vi "verify #frames.vi"(8 "error in (no error)":errorcluster, 11 "Simulated_CCD_Camera in":refnum<class "Sim_Ixon_Ultra.lvclass">) -> (0 "error out":errorcluster, 3 "Simulated_CCD_Camera out":refnum<class "Sim_Ixon_Ultra.lvclass">)   [LabVIEW 2018, in "Sim_Ixon_Ultra.lvclass"]
doc: "Verify the related parameters of the camera\n\nThere are some parameters of the camera operation mode that depend on the value provided for another parameter. This function verifies if these parameters are in agreement."
uses:
  Sim_Ixon_Ultra.lvclass
  <vilib>/ErrorRing/Error Ring.xnode
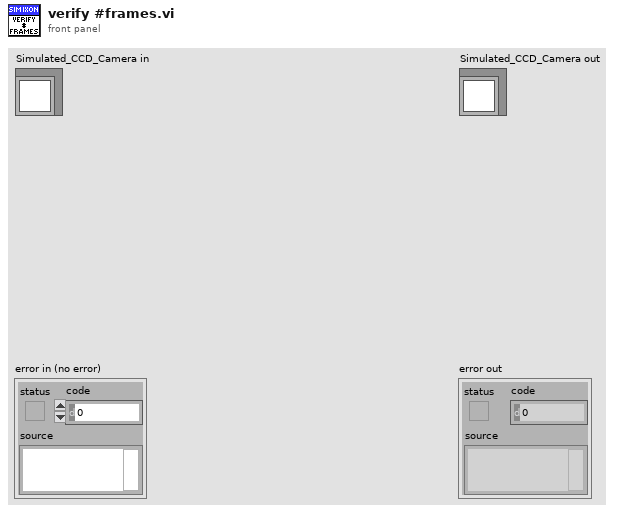
[diagram p1: front panel]
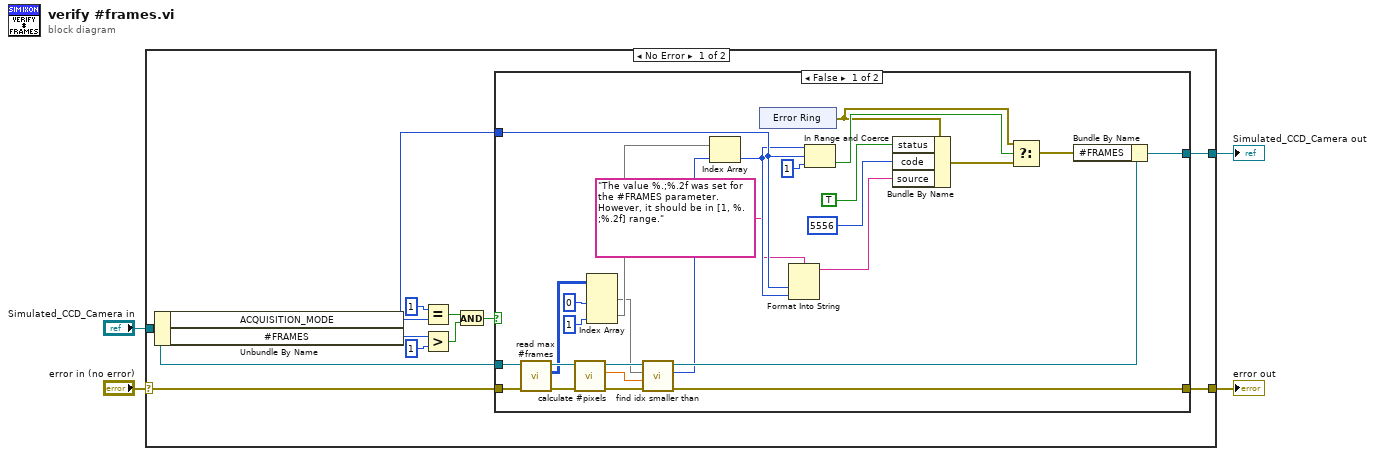
[diagram p0: block diagram]
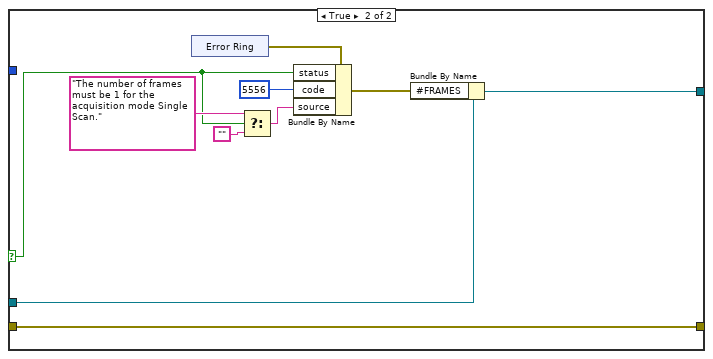
[diagram p2: hidden frame]
diagram:
  n1 = case shown="No Error" "error in (no error)" {
    selector: "error in (no error)" -> [w11 w56]
    tunnel: [w8 w56] -> w3
    tunnel: [w9 w55] -> w1
    tunnel: "Simulated_CCD_Camera in" -> [w10 w55]
    frame No Error {
      n2 = Unbundle By Name(w10) -> ("ACQUISITION_MODE"=w6:u16, "#FRAMES"=w5:u32)
      n3 = Equal?(x=u16 1, y=w6) -> (x = y?=w13:bool)
      n4 = Greater?(x=w5, y=1) -> (0:w14:bool)
      n5 = And(x=w13, y=w14) -> (x .and. y?=w7:bool)
      n6 = case shown="False" w7 {
        selector: w7 -> [_ w44]
        tunnel: [w33 w51] -> w9
        tunnel: w10 -> [w41 w52]
        tunnel: w11 -> [w42 w50]
        tunnel: [w29 w50] -> w8
        tunnel: w5 -> [w32 _]
        frame False {
          n7 = call "read max #frames.vi"("error in (no error)"=w42, "Simulated_CCD_Camera in"=w41) -> ("error out"=w40:errorcluster, "max #pix"=w38:i64[][], "Simulated_CCD_Camera out"=w39:refnum<class "Sim_Ixon_Ultra.lvclass">)  [unwired: 7 in]
          n8 = call "calculate #pixels.vi"("error in (no error)"=w40, "Simulated Camera in"=w39) -> ("error out"=w30:errorcluster, "#pixels"=w25:dbl, "Simulated Camera out"=w27:refnum<class "Sim_Ixon_Ultra.lvclass">)  [unwired: 7 in]
          n9 = Index Array(array=w38, index (col) #1=0 ("disabled index (col)"), index (col) #2=1 ("disabled index (col)")) -> (element #1=w26:i64[], element #2=w35:i64[])  [unwired: 2 in]
          n10 = call "find idx smaller than.vi"("error in (no error)"=w30, "Numeric"=w25, "Array"=w26, "Simulated Camera in"=w27) -> ("error out"=w29:errorcluster, "index"=w24:i32, "Simulated Camera out"=w28:refnum<class "Sim_Ixon_Ultra.lvclass">)  [unwired: 5 in]
          n11 = Index Array(array=w35, index=w24) -> (element=w31:i64)
          n12 = xnode "Error Ring"() -> ("error out"=w16:errorcluster)
          n13 = Format Into String(format string="The value %.;%.2f was set for the #FRAMES parameter. However, it should be in [1, %.;%.2f] range." ("string"), w32, w31) -> (resulting string=w21:string)  [unwired: 2 in, 1 out]
          n14 = In Range and Coerce(upper limit=w31, x=w32, lower limit=1) -> (In Range?=w19:bool)  [unwired: 1 out]
          n15 = Bundle By Name(cluster=w16, "status"=TRUE, "code"=5556, "source"=w21) -> (w17:errorcluster)
          n16 = Select(t=w16, s=w19, f=w17) -> (s? t:f=w18:errorcluster)
          n17 = Bundle By Name(cluster=w28, "#FRAMES"=w18) -> (w33:refnum<class "Sim_Ixon_Ultra.lvclass">)
        }
        frame True {
          n18 = xnode "Error Ring"() -> ("error out"=w53:errorcluster)
          n19 = Select(t="The number of frames must be 1 for the acquisition mode Single Scan.", s=w44, f="") -> (s? t:f=w45:string)
          n20 = Bundle By Name(cluster=w53, "status"=w44, "code"=5556, "source"=w45) -> (w49:errorcluster)
          n21 = Bundle By Name(cluster=w52, "#FRAMES"=w49) -> (w51:refnum<class "Sim_Ixon_Ultra.lvclass">)
        }
      }
    }
    frame Error {
    }
  }
  "error out" <- w3
  "Simulated_CCD_Camera out" <- w1
